vi "Collect Components UI.vi"(8 "error in (no error)":errorcluster, 9 "current component settings":T1[](array[typedef]), 10 "User Interface Handler":refnum<class "User Interface Handler.lvclass">=refnum, 11 "Item Ref in":T2 format="%.0x") -> (0 "error out":errorcluster, 3 "Item Ref out":T2=18446744073709551615 format="%.0x")   [LabVIEW 2019, in "DSF System Explorer.lvlib"]
uses:
  DSF System Explorer.lvlib
  DSF Core.lvlibp/Classes/User Interface/Editors/Component/Component Settings Editor.lvclass
  <vilib>/NI VeriStand/Custom Device API/Custom Device Item Ref.ctl
  <vilib>/NI VeriStand/Custom Device API/Custom Device API.lvlib
  DSF Core.lvlibp/Classes/User Interface Handler/User Interface Handler.lvclass
  DSF Core.lvlibp/Typedefs/DSF Settings Info.ctl
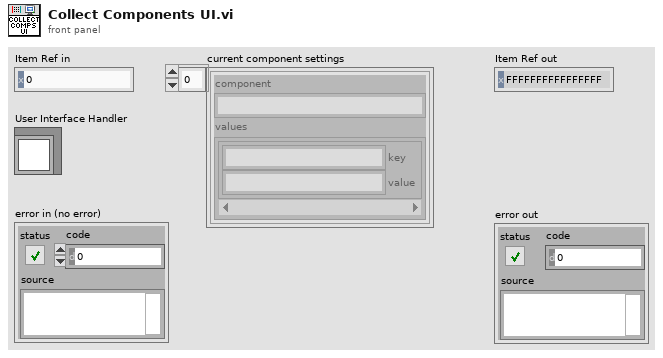
[diagram p1: front panel]
types:
  T1 = typedef "DSF Core.lvlibp/DSF Settings Info.ctl" = cluster{"component":string, "values":cluster{"key":string, "value":string}[]}
  T2 = typedef "Custom Device API.lvlib/Custom Device Item Ref.ctl" = u64
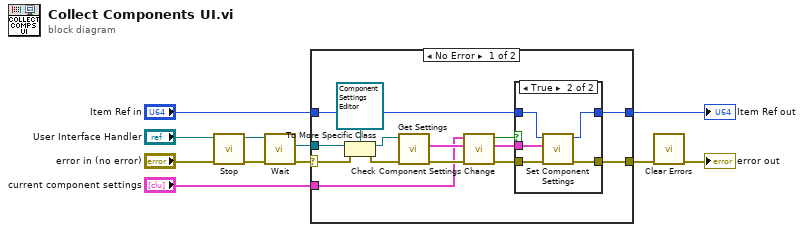
[diagram p0: block diagram]
diagram:
  n1 = call "Stop.vi"("error in (no error)"="error in (no error)", "User Interface Handler in"="User Interface Handler") -> ("error out"=w6:errorcluster, "User Interface Handler out"=w7:refnum<class "User Interface Handler.lvclass">)  [unwired: 8 in]
  n2 = call "Wait.vi"("error in (no error)"=w6, "User Interface Handler in"=w7) -> ("error out"=w9:errorcluster, "User Interface"=w10:refnum<class "User Interface.lvclass">)  [unwired: 7 in, 1 out]
  n3 = case shown="No Error" w9 {
    selector: w9 -> [w23 w33]
    tunnel: w10 -> [w24 _]
    tunnel: "Item Ref in" -> [w21 w34]
    tunnel: [w25 w33] -> w2
    tunnel: [w18 w34] -> w4
    tunnel: "current component settings" -> [w14 _]
    frame No Error {
      n4 = To More Specific Class(target class=refnum<class "Component Settings Editor.lvclass"> refnum ("Component Settings Editor in"), reference=w24, error in=w23) -> (specific class reference=w19:refnum<class "Component Settings Editor.lvclass">, error out=w22:errorcluster)
      n5 = call "Get Settings.vi"("error in (no error)"=w22, "Component Settings Editor in"=w19) -> ("error out"=w17:errorcluster, "component settings"=w16:T1[])  [unwired: 7 in, 1 out]
      n6 = call "Check Component Settings Change.vi"("error in (no error)"=w17, "new component settings"=w16, "current component settings"=w14) -> ("error out"=w12:errorcluster, "new component settings dup"=w15:T1[], "changed?"=w13:bool)  [unwired: 6 in]
      n7 = case shown="True" w13 {
        tunnel: [w27 w32] -> w25
        tunnel: w21 -> [w26 w31]
        tunnel: [w26 w30] -> w18
        tunnel: w15 -> [_ w29]
        tunnel: w12 -> [w27 w28]
        frame False {
        }
        frame True {
          n8 = call "Set Component Settings.vi"("error in (no error)"=w28, "component settings"=w29, "Item Ref in"=w31) -> ("error out"=w32:errorcluster, "Item Ref out"=w30:T2)  [unwired: 7 in]
        }
      }
    }
    frame Error {
    }
  }
  "Item Ref out" <- w4
  n9 = call <vilib>:"Clear Errors.vi"("error in (no error)"=w2) -> ("error out"=→"error out":errorcluster)  [unwired: 5 in, 1 out]
